vi "Initialize Transfer Parameters.vi"(8 "error in (no error)":errorcluster, 10 "Transfer Configurations":T2[](array[typedef]) {"channels"."string offset" format="%d bytes"}, 11 "GE Reflective Memory Transceiver in":refnum<class "GE Reflective Memory Transceiver.lvclass">) -> (0 "error out":errorcluster, 2 "Transfers Parameters":T1[](array[typedef]) {"size" format="%d bytes"; "offset" format="%08x"}, 3 "GE Reflective Memory Transceiver out":refnum<class "GE Reflective Memory Transceiver.lvclass">)   [LabVIEW 2017, in "GE Reflective Memory Transceiver.lvlib" / "GE Reflective Memory Transceiver.lvclass"]
uses:
  GE Reflective Memory Transceiver.lvclass
  Builds/Data Sharing Framework/Current/Core/DSF Core.lvlibp/Typedefs/DSF Engine Transfer Configuration.ctl
  Builds/Data Sharing Framework/Current/Core/DSF Core.lvlibp/Typedefs/DSF Byte Order.ctl
  Builds/Data Sharing Framework/Current/Core/DSF Core.lvlibp/Typedefs/DSF Settings Info.ctl
  Builds/Data Sharing Framework/Current/Core/DSF Core.lvlibp/Typedefs/DSF Engine Channel Configuration.ctl
  Builds/Data Sharing Framework/Current/Core/DSF Core.lvlibp/Typedefs/DSF Data Type.ctl
  Transfer Parameters.ctl
  Transfer Buffer.ctl
  GE Reflective Memory Transceiver.lvclass/GE Reflective Memory Transceiver.ctl
  Builds/Data Sharing Framework/Current/Core/DSF Core.lvlibp/Classes/Configuration/Required Buffer Size (Transfer).vi
  Builds/Data Sharing Framework/Current/Core/DSF Core.lvlibp/Classes/Configuration/Configuration Session.lvclass
  Builds/Data Sharing Framework/Current/Core/DSF Core.lvlibp
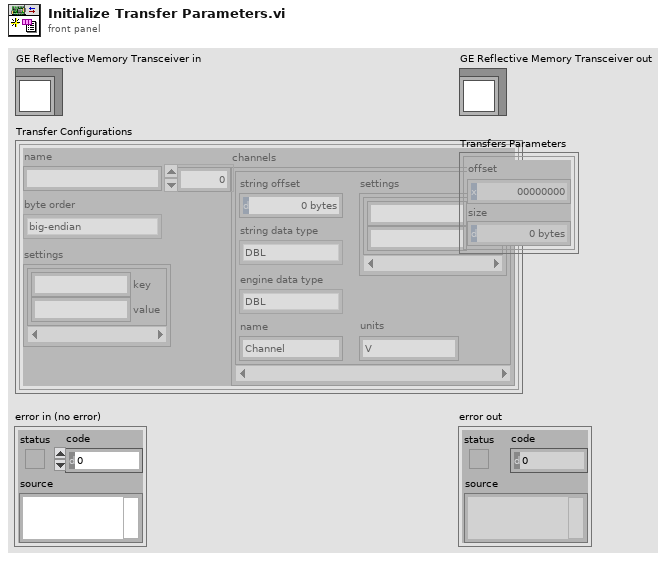
[diagram p1: front panel]
types:
  T1 = typedef "GE Reflective Memory Transceiver.lvlib/GE Reflective Memory Transceiver.lvclass/Transfer Parameters.ctl" = cluster{"offset":u32, "size":u32}
  T2 = typedef "DSF Core.lvlibp/DSF Engine Transfer Configuration.ctl" = cluster{"name":string, "byte order":T3, "settings":T4, "channels":T5[]}
  T3 = typedef "DSF Core.lvlibp/DSF Byte Order.ctl" = enum8{"big-endian", "little-endian"}
  T4 = typedef "DSF Core.lvlibp/DSF Settings Info.ctl" = cluster{"key":string, "value":string}[]
  T5 = typedef "DSF Core.lvlibp/DSF Engine Channel Configuration.ctl" = cluster{"string offset":u64, "string data type":T6, "engine data type":T6, "name":string, "settings":T4, "units":string}
  T6 = typedef "DSF Core.lvlibp/DSF Data Type.ctl" = enum8{"Bool", "SGL", "DBL", "I8", "I16", "I32", "I64", "U8", "U16", "U32", "U64"}
  T7 = typedef "GE Reflective Memory Transceiver.lvlib/GE Reflective Memory Transceiver.lvclass/Transfer Buffer.ctl" = enum16{"Engine", "String"}
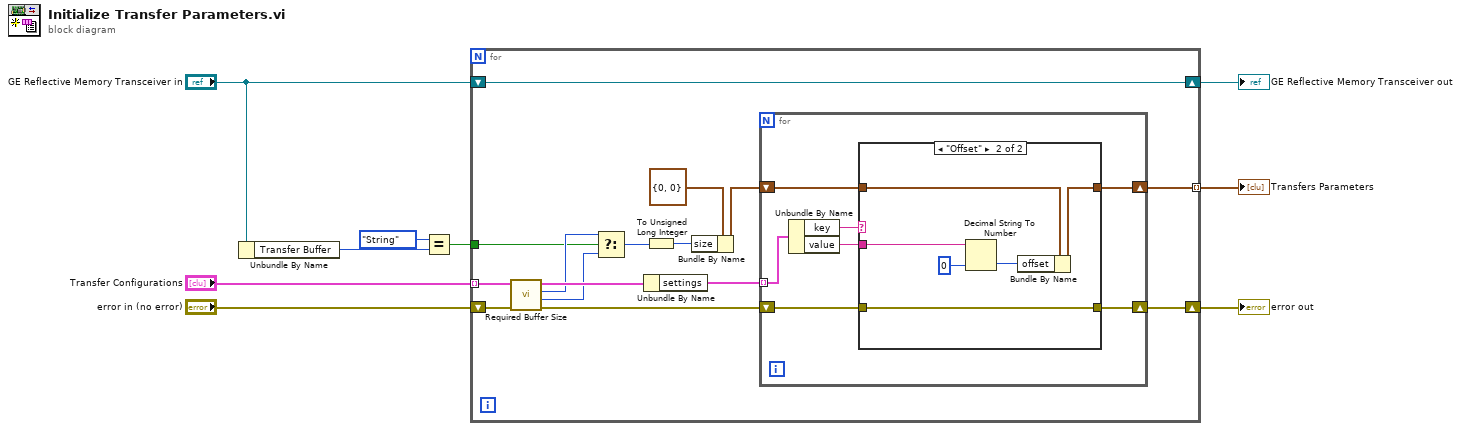
[diagram p0: block diagram]
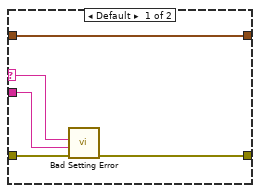
[diagram p2: hidden frame]
diagram:
  n1 = Unbundle By Name("GE Reflective Memory Transceiver in") -> ("Transfer Buffer"=w3:T7)
  n2 = Equal?(x=Transfer_Buffer."String", y=w3) -> (x = y?=w1:bool)
  n3 = for {
    shift-right: [w17] -> w7
    shift-left: "error in (no error)" -> [w24]
    tunnel: "Transfer Configurations" -> [w16] mode=indexing
    shift-right: [w19] -> w9
    shift-left: "GE Reflective Memory Transceiver in" -> [w19]
    tunnel: [w18] -> w5 mode=indexing
    tunnel: w1 -> [w10]
    n4 = call-poly "Required Buffer Size.vi"("error in (no error)"=w24, "Transfer Configuration in"=w16) -> ("error out"=w21:errorcluster, "engine buffer size"=w13:u64, "string buffer size"=w12:u64, "Transfer Configuration out"=w15:T2)  [unwired: 6 in]
    n5 = Select(t=w12, s=w10, f=w13) -> (s? t:f=w11:u64)
    n6 = Unbundle By Name(w15) -> ("settings"=w14:T4)
    n7 = To Unsigned Long Integer(number=w11) -> (unsigned 32bit integer=w22:u32)
    n8 = Bundle By Name(cluster=T1 {"offset"=0, "size"=0} ("Transfer Parameters"), "size"=w22) -> (w23:T1)
    n9 = for {
      shift-right: [w25] -> w17
      shift-left: w21 -> [w31]
      tunnel: w14 -> [w30] mode=indexing
      shift-right: [w26] -> w18
      shift-left: w23 -> [w28]
      n10 = Unbundle By Name(w30) -> ("key"=w29:string, "value"=w27:string)
      n11 = case shown="\"Offset\"" w29 {
        selector: w29 -> [w33 _]
        tunnel: w31 -> [w35 w37]
        tunnel: w28 -> [w36 w42]
        tunnel: w27 -> [w34 w40]
        tunnel: [w36 w41] -> w26
        tunnel: [w32 w37] -> w25
        frame Default {
          n12 = call "Bad Setting Error.vi"("error in (no error)"=w35, "value"=w34, "key"=w33) -> ("error out"=w32:errorcluster)  [unwired: 7 in, 1 out]
        }
        frame "Offset" {
          n13 = Decimal String To Number(string=w40, default (0L)=u32 0 ("default (0 I32)")) -> (number=w39:u32)  [unwired: 1 in, 1 out]
          n14 = Bundle By Name(cluster=w42, "offset"=w39) -> (w41:T1)
        }
      }
    }
  }
  "error out" <- w7
  "GE Reflective Memory Transceiver out" <- w9
  "Transfers Parameters" <- w5
